vi "povorot_posle_zahvata.vi"() -> ()   [LabVIEW 2017]
uses:
  <vilib>/userdefined/High Color/IMAQdx.ctl
  <vilib>/vision/driver/NI_Vision_Acquisition_Software.lvlib
panel:
  out "X":sgl
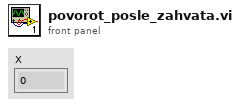
[diagram p1: front panel]
types:
  T1 = typedef "IMAQdx.ctl" = refnum<k21>
  T2 = typedef "IMAQ Image.ctl" = refnum<image>
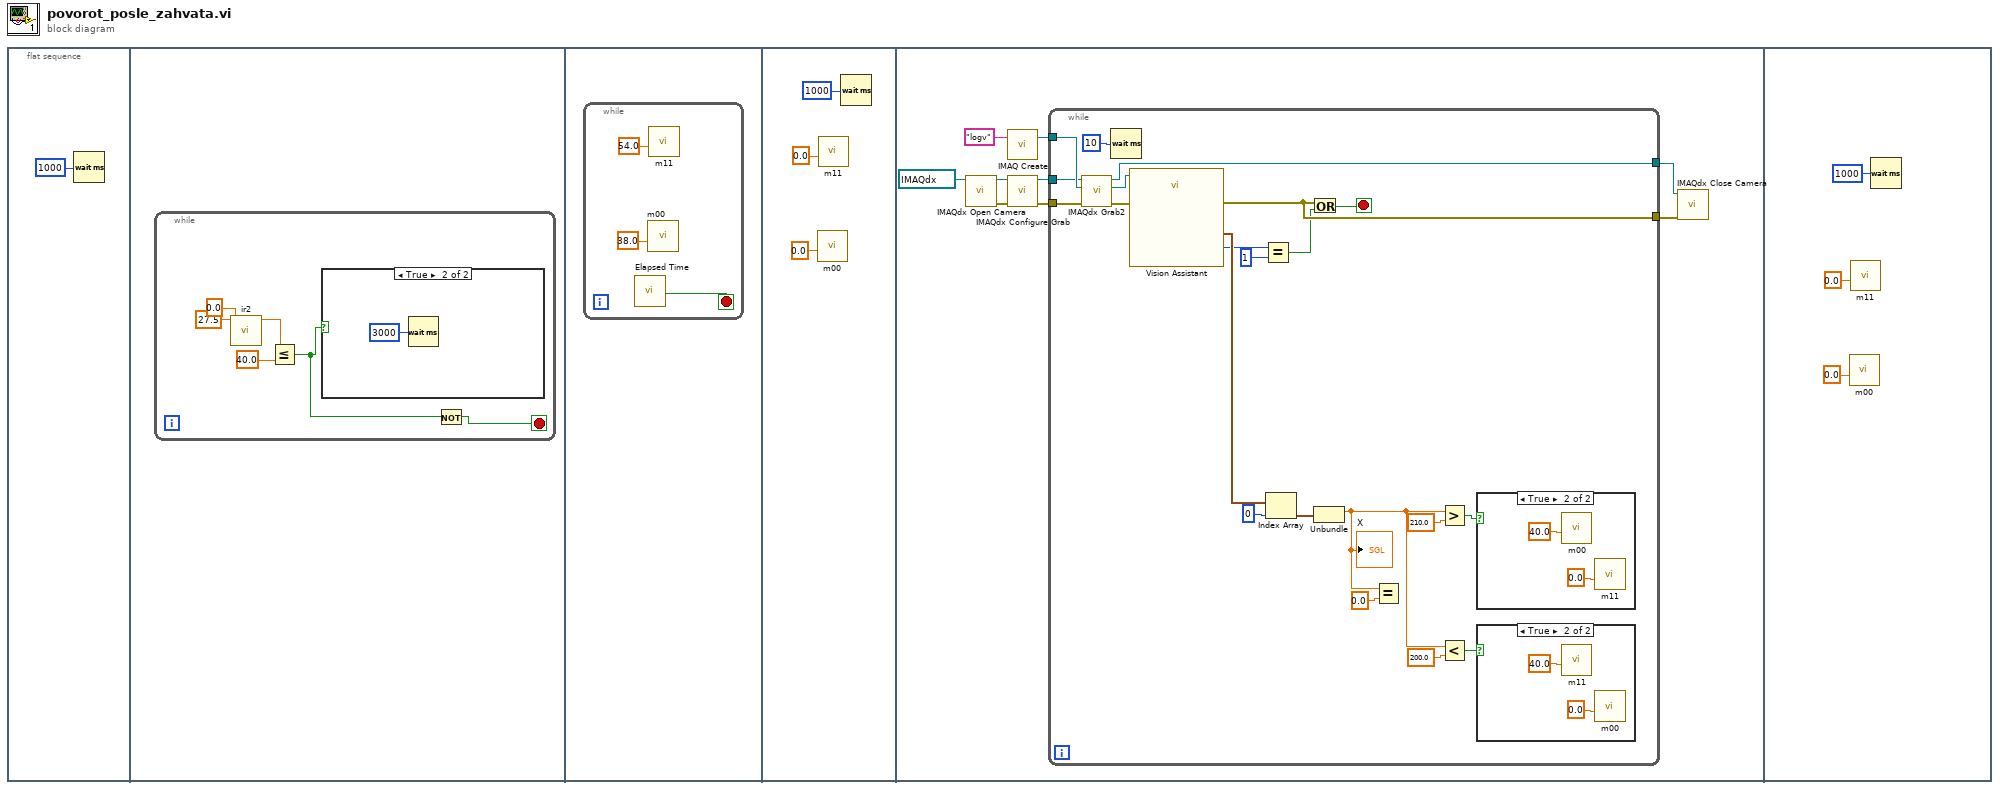
[diagram p0: block diagram]
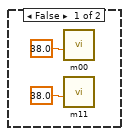
[diagram p3: hidden frame]
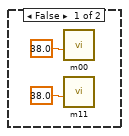
[diagram p4: hidden frame]
diagram:
  n1 = flat-sequence {
    frame #0 {
      n2 = Wait (ms)(milliseconds to wait=u32 1000) -> ()  [unwired: 1 out]
    }
    frame #1 {
      n3 = while {
        stop <- w3 stop-if-true
        n4 = call "ir2.vi"("Koffset [cm]"=0.0, "Kscale [cm-V]"=27.5) -> ("см"=w5:dbl)  [unwired: 8 in, 1 out]
        n5 = Less Or Equal?(x=w5, y=40.0) -> (x <= y?=w2:bool)
        n6 = case shown="True" w2 {
          frame False {
          }
          frame True {
            n7 = Wait (ms)(milliseconds to wait=u32 3000) -> ()  [unwired: 1 out]
          }
        }
        n8 = Not(x=w2) -> (.not. x?=w3:bool)
      }
    }
    frame #2 {
      n9 = while {
        stop <- w9 stop-if-true
        n10 = call "Elapsed Time"() -> ("Time has Elapsed"=w9:bool)  [unwired: 12 in, 7 out]
        n11 = call "m00.vi"("position"=38.0) -> ()  [unwired: 10 in, 1 out]
        n12 = call "m11.vi"("position"=54.0) -> ()  [unwired: 10 in, 1 out]
      }
    }
    frame #3 {
      n13 = call "m00.vi"("position"=0.0) -> ()  [unwired: 10 in, 1 out]
      n14 = call "m11.vi"("position"=0.0) -> ()  [unwired: 10 in, 1 out]
      n15 = Wait (ms)(milliseconds to wait=u32 1000) -> ()  [unwired: 1 out]
    }
    frame #4 {
      n16 = call <vilib>:"IMAQdx Open Camera.vi"("Session In"=T1 "cam1") -> ("error out"=w20:errorcluster, "Session Out"=w19:T1)  [unwired: 9 in]
      n17 = call "IMAQ Create"("Image Name"="logv") -> ("New Image"=w17:T2)  [unwired: 4 in, 1 out]
      n18 = call <vilib>:"IMAQdx Configure Grab.vi"("error in"=w20, "Session In"=w19) -> ("error out"=w21:errorcluster, "Session Out"=w18:T1)  [unwired: 8 in]
      n19 = while {
        tunnel: w21 -> [w39]
        tunnel: w17 -> [w38]
        tunnel: w18 -> [w37]
        tunnel: [w36] -> w23
        tunnel: [w34] -> w22
        stop <- w35 stop-if-true
        n20 = call <vilib>:"IMAQdx Grab2.vi"("error in"=w39, "Image In"=w38, "Session In"=w37) -> ("error out"=w41:errorcluster, "Image Out"=w40:T2, "Session Out"=w36:T1)  [unwired: 5 in, 1 out]
        n21 = Wait (ms)(milliseconds to wait=u32 10) -> ()  [unwired: 1 out]
        n22 = call "Vision Assistant"("Image In"=w40, "error in"=w41) -> ("Edges Coordinates (Edge Detector 1)"=w44:cluster{"X":sgl, "Y":sgl}[], "Number of Matches (Color Location 1)"=w26:i32, "error out"=w34:errorcluster)  [unwired: 22 in, 1 out]
        n23 = Equal?(x=w26, y=1) -> (x = y?=w25:bool)
        n24 = Index Array(array=w44, index=0) -> (element=w43:cluster{"X":sgl, "Y":sgl})
        n25 = Or(x=w34, y=w25) -> (x .or. y?=w35:bool)
        n26 = Unbundle(w43) -> ("X"=w29:sgl)  [unwired: 1 out]
        "X" <- w29
        n27 = Equal?(x=w29, y=sgl 0.0) -> ()  [unwired: 1 out]
        n28 = Greater?(x=w29, y=sgl 210.0) -> (0:w32:bool)
        n29 = Less?(x=w29, y=sgl 200.0) -> (x < y?=w28:bool)
        n30 = case shown="True" w32 {
          frame False {
            n31 = call "m00.vi"("position"=38.0) -> ()  [unwired: 10 in, 1 out]
            n32 = call "m11.vi"("position"=38.0) -> ()  [unwired: 10 in, 1 out]
          }
          frame True {
            n33 = call "m00.vi"("position"=40.0) -> ()  [unwired: 10 in, 1 out]
            n34 = call "m11.vi"("position"=0.0) -> ()  [unwired: 10 in, 1 out]
          }
        }
        n35 = case shown="True" w28 {
          frame False {
            n36 = call "m00.vi"("position"=38.0) -> ()  [unwired: 10 in, 1 out]
            n37 = call "m11.vi"("position"=38.0) -> ()  [unwired: 10 in, 1 out]
          }
          frame True {
            n38 = call "m11.vi"("position"=40.0) -> ()  [unwired: 10 in, 1 out]
            n39 = call "m00.vi"("position"=0.0) -> ()  [unwired: 10 in, 1 out]
          }
        }
      }
      n40 = call <vilib>:"IMAQdx Close Camera.vi"("error in"=w22, "Session In"=w23) -> ()  [unwired: 9 in, 1 out]
    }
    frame #5 {
      n41 = call "m00.vi"("position"=0.0) -> ()  [unwired: 10 in, 1 out]
      n42 = call "m11.vi"("position"=0.0) -> ()  [unwired: 10 in, 1 out]
      n43 = Wait (ms)(milliseconds to wait=u32 1000) -> ()  [unwired: 1 out]
    }
  }
